vi "Set Period.vi"(6 "Pump Name":string="Message Pump", 8 "error in":errorcluster, 10 "Period in ms (-1)":i32=-1, 11 "Worker":refnum<class "Worker.lvclass">) -> (0 "error out":errorcluster, 3 "Worker out":refnum<class "Worker.lvclass">)   [LabVIEW 2021, in "Message Pump.lvclass"]
doc: "Sets the duration time in milliseconds between pumped messages. 20 ms is the minimum possible duration. A value of -1 will stop messages from being pumped.\n\nThis VI returns an error if the Message Pump, as identified through <b>Pump Name</b> is not found to exist.\n\n-----------\n\n<b>Inputs ></b>\n\n<b>Period (ms)</b>: The time duration (in ms) between each pumped message. 20 ms is the minimum possible duration. A value of -1 will stop messages from being pumped.\n\n<b>Pump Name</b>: The name of the message pump. This name is local to the Worker it is called from. This input is required if multiple Message Pumps are to be used by the calling Worker."
uses:
  Message Pump.lvclass
  <vilib>/addons/_Workers/Library/Classes/Worker/Worker.lvclass
  <vilib>/addons/_Workers/Library/Classes/Worker/Worker.lvclass/Worker.ctl
  <vilib>/addons/_Workers/Library/Classes/Worker/Find subWorker Queue from Alias.vi
  <vilib>/addons/_Workers/Library/Classes/Worker/Read subWorker Data.vi
  <vilib>/Utility/error.llb/Clear Errors.vi
  <vilib>/Utility/error.llb/Error Cluster From Error Code.vi
  <vilib>/addons/_Workers/Library/Classes/Message/Enqueue Message to Queue.vi
  <vilib>/addons/_Workers/Library/Classes/Message/Message.lvclass
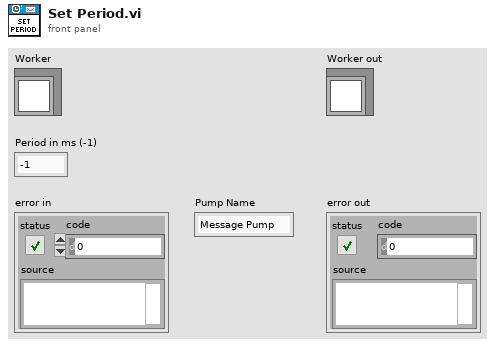
[diagram p1: front panel]
types:
  T1 = typedef "WORKERS.lvlib/Case Label.ctl" = string
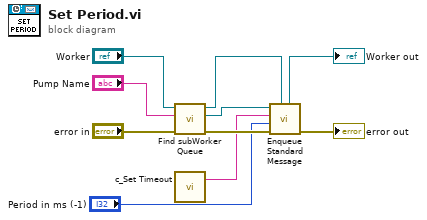
[diagram p0: block diagram]
diagram:
  n1 = call-poly <vilib>:"Find subWorker Queue.vi"("error in"="error in", "subWorker Alias"="Pump Name", "Worker"="Worker") -> ("error out"=w10:errorcluster, "Message Queue"=w1:refnum<class "Message Queue.lvclass">, "dup Worker out"=w4:refnum<class "Worker.lvclass">)  [unwired: 6 in]
  n2 = call "c_Set Timeout.vi"() -> ("Case Label"=w8:T1)  [unwired: 1 in]
  n3 = call-poly <vilib>:"Enqueue Standard Message.vi"("Worker"=w4, "error in"=w10, "Data"="Period in ms (-1)", "Case Label"=w8, "Message Queue"=w1) -> ("error out"=→"error out":errorcluster, "dup Worker out"=→"Worker out":refnum<class "Worker.lvclass">)  [unwired: 4 in, 1 out]
